vi "Build Pkg Directory.vi"(11 "error in (no error)":errorcluster) -> (4 "Path":path, 15 "error out":errorcluster)   [LabVIEW 2021, in "Measurement Builder.lvlib"]
uses:
  Measurement Builder.lvlib
  Dictionary/Dictionary.lvlib
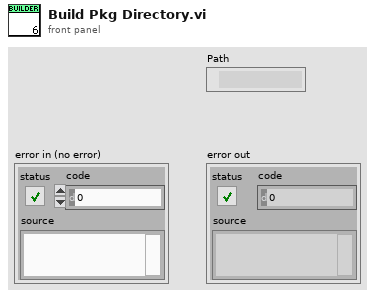
[diagram p1: front panel]
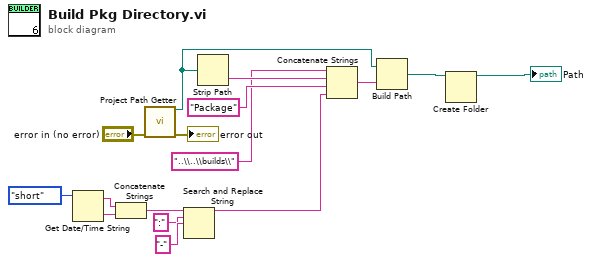
[diagram p0: block diagram]
diagram:
  n1 = Get Date/Time String(date format (0)=enum16{"short", "long", "abbreviated"}."short") -> (date string=w11:string, time string=w12:string)  [unwired: 2 in]
  n2 = Concatenate Strings(w11, w12) -> (w13:string)
  n3 = call "Project Path Getter.vi"("error in (no error)"="error in (no error)") -> ("Path"=w7:path, "error out"=→"error out":errorcluster)  [unwired: 13 in]
  n4 = Search and Replace String(input string=w13, search string=":", replace string="-" ("replace string (\"\")")) -> (result string=w3:string)  [unwired: 5 in, 3 out]
  n5 = Strip Path(path=w7) -> (name=w9:string)  [unwired: 1 out]
  n6 = Concatenate Strings("..\\..\\builds\\" ("string"), w9, "Package" ("string"), w3) -> (w4:string)
  n7 = Build Path(base path=w7, name or relative path=w4) -> (appended path=w2:path)
  n8 = Create Folder(path (use dialog)=w2) -> (created path=→"Path":path)  [unwired: 2 in, 2 out]
